vi "Home Dialog.vi"(8 "error in (no error)":errorcluster) -> (0 "error out":errorcluster)   [LabVIEW 2014, in "Raspberry Pi Compatible Compiler for LabVIEW.lvlib"]
doc: "Home version license dialog."
uses:
  Raspberry Pi Compatible Compiler for LabVIEW.lvlib
panel:
  in  "OK":bool
  # "You are using the Raspberry Pi Compatible Compiler for LabVIEW Home Edition.  This edition is for Home or Student use ONLY.  You must upgrade to the Standard Edition if being used in a professional setting according to the license agreement.\n\nBy acknowledging this message, you agree to the terms bound by the Arduino Compatible Compiler for LabVIEW Home Edition license agreement."
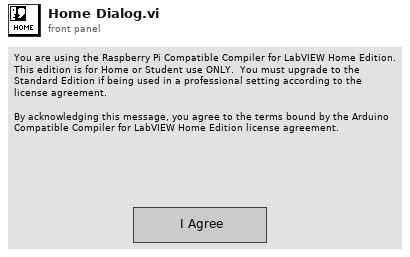
[diagram p1: front panel]
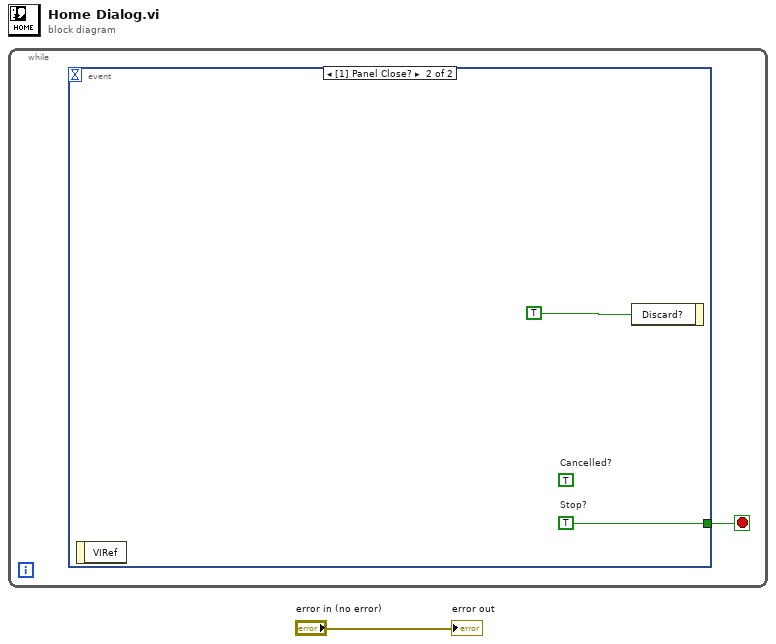
[diagram p0: block diagram]
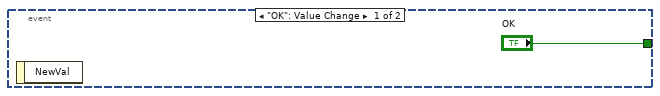
[diagram p2: hidden frame]
diagram:
  n1 = while {
    stop <- w2 stop-if-true
    n2 = event shown="[1] Panel Close?" {
      selector: _ -> [_ _]
      dyn-events: _ -> [_ _]
      timeout: _ -> [_ _]
      tunnel: ["OK" w4] -> w2
      event "OK": Value Change {
        n3 = event-data() -> ()  [unwired: 1 in, 1 out]
      }
      event Panel Close? {
        (unwired) TRUE  # Cancelled?
        w4 = TRUE  # Stop?
        n4 = event-data() -> ()  [unwired: 1 in, 1 out]
        n5 = event-data("Discard?"=TRUE) -> ()  [unwired: 1 in, 1 out]
      }
    }
  }
  "error out" <- "error in (no error)"
